vi "Se Confirm Color.vi"() -> ()   [LabVIEW 2012]
panel:
  in  "Colors [4] 2":cluster{u32, u32}[](array[cluster])
  in  "Gray OFF/Red ON":bool
  out "Numeric":u32 format="%#_9g"
  in  "Color Box":u32(colorbox)
  out "element":cluster{"Color Box":u32, "Color Box":u32}
  in  "Colors [4]":cluster{u32, u32}[](array[cluster])
  in  "Confirm Now":bool
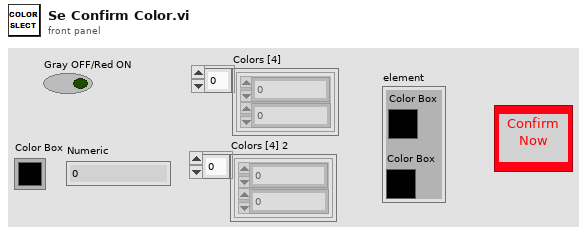
[diagram p1: front panel]
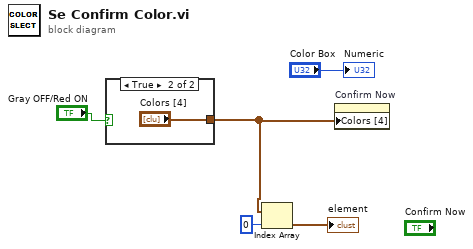
[diagram p0: block diagram]
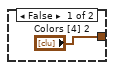
[diagram p2: hidden frame]
diagram:
  n1 = case shown="True" "Gray OFF/Red ON" {
    tunnel: ["Colors [4] 2" "Colors [4]"] -> w5
    frame False {
    }
    frame True {
    }
  }
  n2 = Index Array(array=w5, index=0) -> (element=→"element":cluster{u32, u32})
  n3 = property on="Confirm Now" class="Bool (strict)"("Colors [4]"=w5) -> ()  [unwired: 2 in, 2 out]
  "Numeric" <- "Color Box"
